vi "DisplaySequenceFile Event Callback.vi"(4 "SequenceFile View Manager":refnum<k7>, 5 "Event data":cluster{"file":refnum<k7>, "reason":i32}, 6 "CtlRef":refnum<k7>, 7 "Event common data":cluster{"Source":i32, "Type":u32, "Time":u32}) -> ()   [LabVIEW 2010, in "TS Simple LabVIEW OI Dependencies.lvlib"]
uses:
  TS Simple LabVIEW OI Dependencies.lvlib
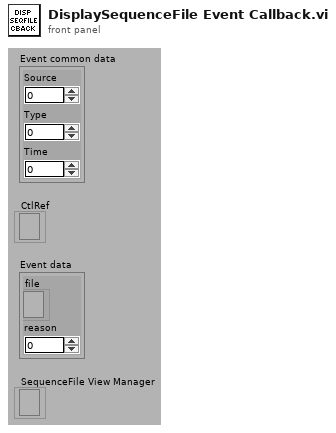
[diagram p1: front panel]
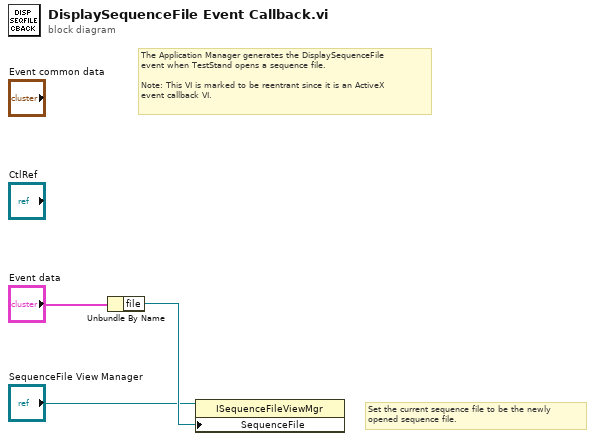
[diagram p0: block diagram]
diagram:
  # "Set the current sequence file to be the newly\nopened sequence file."
  # "The Application Manager generates the DisplaySequenceFile\nevent when TestStand opens a sequence file.\n\nNote: This VI is marked to be reentrant since it is an ActiveX\nevent callback VI."
  n1 = Unbundle By Name("Event data") -> ("file"=w3:refnum<k7>)
  n2 = property class="ISequenceFileViewMgr"(reference="SequenceFile View Manager", "SequenceFile"=w3) -> ()  [unwired: 1 in, 2 out]
